vi "xps_panel_DO_disconnect_from_controller.vi"(8 "error in (no error)":errorcluster, 11 "newport_xps_panel in":refnum<class "newport_xps_panel.lvclass">) -> (0 "error out":errorcluster, 3 "newport_xps_panel out":refnum<class "newport_xps_panel.lvclass">)   [LabVIEW 2015, in "newport_xps_panel.lvclass"]
uses:
  newport_xps_panel.lvclass
  newport_xps/newport_xps.lvclass
  UI/panel_class/panel.lvclass
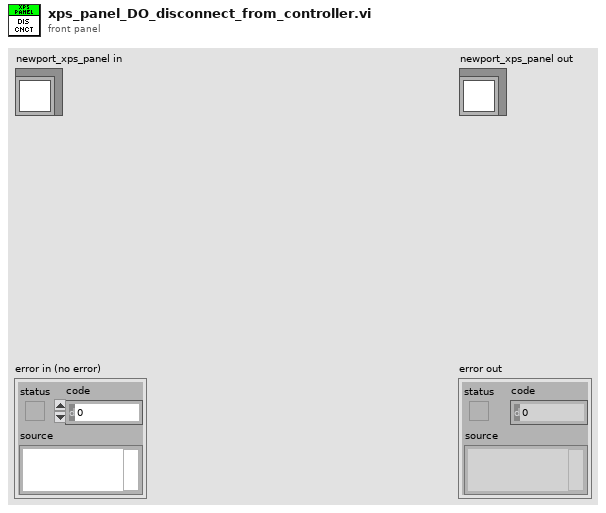
[diagram p1: front panel]
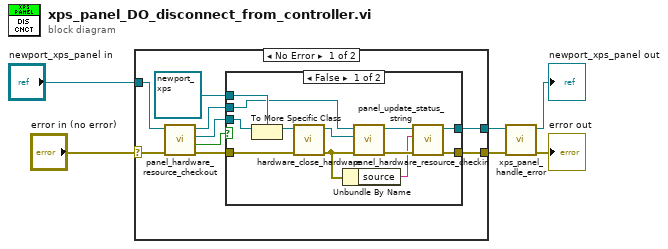
[diagram p0: block diagram]
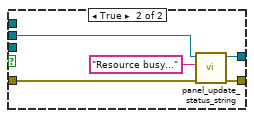
[diagram p2: hidden frame]
diagram:
  n1 = case shown="No Error" "error in (no error)" {
    selector: "error in (no error)" -> [w15 w34]
    tunnel: [w9 w34] -> w4
    tunnel: [w8 w33] -> w2
    tunnel: "newport_xps_panel in" -> [w14 w33]
    frame No Error {
      n2 = call "panel_hardware_resource_checkout.vi"("error in (no error)"=w15, "panel in"=w14) -> ("error out"=w10:errorcluster, "timed out?"=w13:bool, "hardware.lvclass"=w11:refnum<class "hardware.lvclass">, "panel out"=w12:refnum<class "newport_xps_panel.lvclass">)  [unwired: 6 in]
      n3 = case shown="False" w13 {
        tunnel: w12 -> [w23 w29]
        tunnel: w11 -> [w25 _]
        tunnel: w10 -> [w22 w32]
        tunnel: [w17 w31] -> w9
        tunnel: [w16 w28] -> w8
        tunnel: refnum<class "newport_xps.lvclass"> refnum ("newport_xps in") -> [w24 _]
        frame False {
          n4 = To More Specific Class(target class=w24, reference=w25) -> (specific class reference=w21:refnum<class "newport_xps.lvclass">)  [unwired: 1 in, 1 out]
          n5 = call-dynamic "hardware_close_hardware.vi"("error in (no error)"=w22, "newport_xps in"=w21) -> ("error out"=w19:errorcluster, "newport_xps out"=w20:refnum<class "newport_xps.lvclass">)  [unwired: 8 in]
          n6 = Unbundle By Name(w19) -> ("source"=w18:string)
          n7 = call "panel_hardware_resource_checkin.vi"("error in (no error)"=w19, "hardware.lvclass"=w20, "panel in"=w23) -> ("error out"=w26:errorcluster, "panel out"=w27:refnum<class "newport_xps_panel.lvclass">)  [unwired: 7 in]
          n8 = call-dynamic "panel_update_status_string.vi"("error in (no error)"=w26, "String"=w18, "newport_xps_panel in"=w27) -> ("error out"=w17:errorcluster, "newport_xps_panel out"=w16:refnum<class "newport_xps_panel.lvclass">)  [unwired: 7 in]
        }
        frame True {
          n9 = call-dynamic "panel_update_status_string.vi"("error in (no error)"=w32, "String"="Resource busy...", "newport_xps_panel in"=w29) -> ("error out"=w31:errorcluster, "newport_xps_panel out"=w28:refnum<class "newport_xps_panel.lvclass">)  [unwired: 7 in]
        }
      }
    }
    frame Error {
    }
  }
  n10 = call "xps_panel_handle_error.vi"("error in (no error)"=w4, "newport_xps_panel in"=w2) -> ("error out"=→"error out":errorcluster, "newport_xps_panel out"=→"newport_xps_panel out":refnum<class "newport_xps_panel.lvclass">)  [unwired: 8 in]
